vi "行删除.vi"(8 "error in (no error)":errorcluster caption="错误输入（无错误）", 11 "程序 输入":refnum<class "程序.lvclass">) -> (0 "error out":errorcluster caption="错误输出", 3 "程序 输出":refnum<class "程序.lvclass">)   [LabVIEW 2020, in "程序.lvclass"]
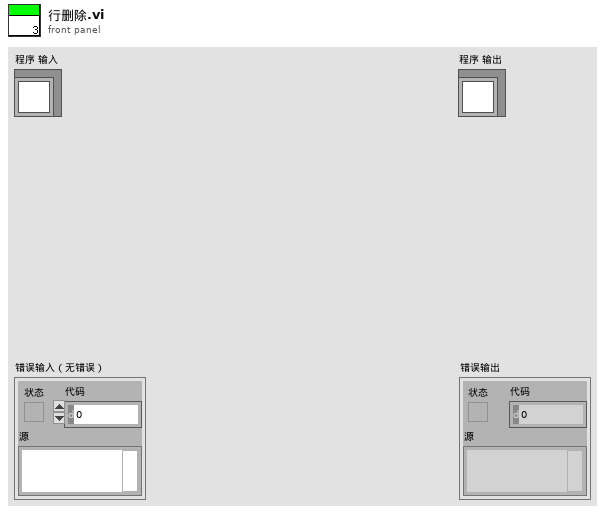
[diagram p1: front panel]
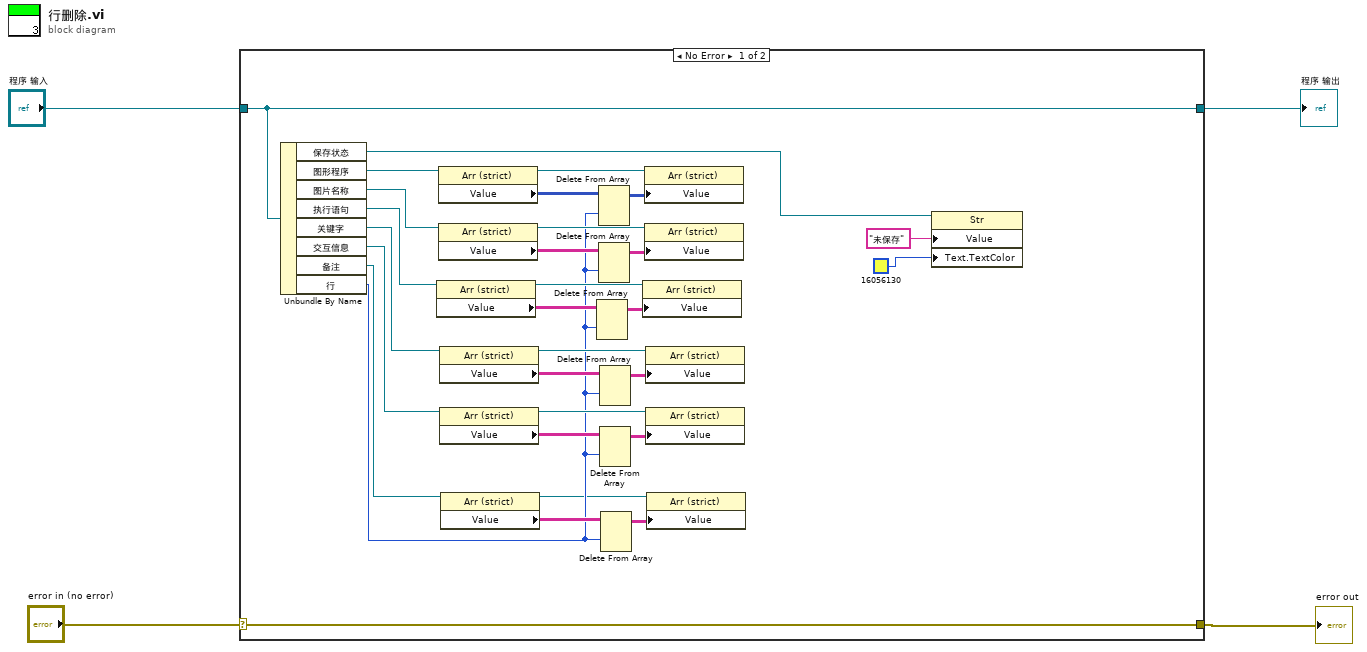
[diagram p0: block diagram]
diagram:
  n1 = case shown="No Error" "error in (no error)" {
    selector: "error in (no error)" -> [w34 w36]
    tunnel: [w34 w36] -> w2
    tunnel: [w33 w35] -> w3
    tunnel: "程序 输入" -> [w33 w35]
    frame No Error {
      n2 = Unbundle By Name(w33) -> ("保存状态"=w10:refnum<vi>, "图形程序"=w32:refnum<vi>, "图片名称"=w25:refnum<vi>, "执行语句"=w21:refnum<vi>, "关键字"=w18:refnum<vi>, "交互信息"=w13:refnum<vi>, "备注"=w6:refnum<vi>, "行"=w7:u32)
      n3 = property class="Arr (strict)"(reference=w21) -> (reference out=w22:refnum<vi>, "Value"=w23:string[][])  [unwired: 1 in, 1 out]
      n4 = property class="Arr (strict)"(reference=w32) -> (reference out=w31:refnum<vi>, "Value"=w30:picture[][])  [unwired: 1 in, 1 out]
      n5 = property class="Arr (strict)"(reference=w25) -> (reference out=w26:refnum<vi>, "Value"=w27:string[][])  [unwired: 1 in, 1 out]
      n6 = property class="Arr (strict)"(reference=w18) -> (reference out=w17:refnum<vi>, "Value"=w20:string[][])  [unwired: 1 in, 1 out]
      n7 = property class="Arr (strict)"(reference=w13) -> (reference out=w16:refnum<vi>, "Value"=w14:string[][])  [unwired: 1 in, 1 out]
      n8 = property class="Arr (strict)"(reference=w6) -> (reference out=w5:refnum<vi>, "Value"=w9:string[][])  [unwired: 1 in, 1 out]
      n9 = Delete From Array(array=w23, index (row)=w7) -> (array with subset deleted=w24:string[][])  [unwired: 2 in, 1 out]
      n10 = Delete From Array(array=w30, index (row)=w7) -> (array with subset deleted=w29:picture[][])  [unwired: 2 in, 1 out]
      n11 = Delete From Array(array=w27, index (row)=w7) -> (array with subset deleted=w28:string[][])  [unwired: 2 in, 1 out]
      n12 = Delete From Array(array=w20, index (row)=w7) -> (array with subset deleted=w19:string[][])  [unwired: 2 in, 1 out]
      n13 = Delete From Array(array=w14, index (row)=w7) -> (array with subset deleted=w15:string[][])  [unwired: 2 in, 1 out]
      n14 = Delete From Array(array=w9, index (row)=w7) -> (array with subset deleted=w8:string[][])  [unwired: 2 in, 1 out]
      n15 = property class="Arr (strict)"(reference=w22, "Value"=w24) -> ()  [unwired: 1 in, 2 out]
      n16 = property class="Arr (strict)"(reference=w31, "Value"=w29) -> ()  [unwired: 1 in, 2 out]
      n17 = property class="Arr (strict)"(reference=w26, "Value"=w28) -> ()  [unwired: 1 in, 2 out]
      n18 = property class="Arr (strict)"(reference=w17, "Value"=w19) -> ()  [unwired: 1 in, 2 out]
      n19 = property class="Arr (strict)"(reference=w16, "Value"=w15) -> ()  [unwired: 1 in, 2 out]
      n20 = property class="Arr (strict)"(reference=w5, "Value"=w8) -> ()  [unwired: 1 in, 2 out]
      n21 = property class="Str"(reference=w10, "Value"="未保存" ("值"), "Text.TextColor"=u32 16056130) -> ()  [unwired: 1 in, 2 out]
    }
    frame Error {
    }
  }
  "error out" <- w2
  "程序 输出" <- w3
